vi "Validate.vi"(1 "Path":path) -> (0 "Shortcut or not a path?":bool)   [LabVIEW 2011]
doc: "This VI checks if the path selected is a shortcut or Not a Path. These directories will not be considered in the tree control."
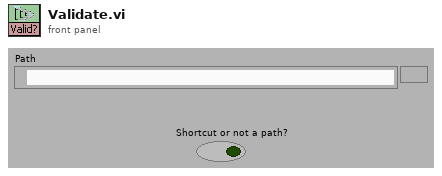
[diagram p1: front panel]
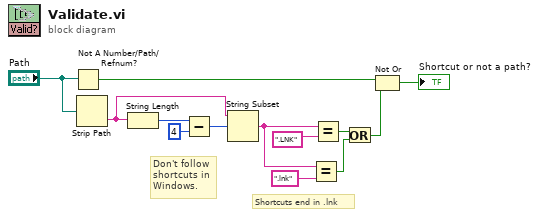
[diagram p0: block diagram]
diagram:
  # "Shortcuts end in .lnk"
  # "Don't follow shortcuts in Windows."
  n1 = Not A Number/Path/Refnum?(number/path/refnum="Path") -> (NaN/Path/Refnum?=w8:bool)
  n2 = Strip Path(path="Path") -> (name=w2:string)  [unwired: 1 out]
  n3 = String Length(string=w2) -> (length=w3:i32)
  n4 = Subtract(x=w3, y=4) -> (x-y=w5:i32)
  n5 = String Subset(string=w2, offset (0)=w5) -> (substring=w10:string)  [unwired: 1 in]
  n6 = Equal?(x=w10, y=".lnk") -> (x = y?=w11:bool)
  n7 = Equal?(x=w10, y=".LNK") -> (x = y?=w9:bool)
  n8 = Or(x=w9, y=w11) -> (x .or. y?=w12:bool)
  n9 = Not Or(1:w12, 2:w8) -> (0:→"Shortcut or not a path?":bool)
